vi "main.vi"(0 "Test Pins":T7, 1 "Caller Information":T11, 5 "Test Inputs":T8={"Load Current in A"=0.0, "Input Voltage in V"=[], "Nominal Output Voltage in V"=0.0, "Required Vout drop"=0.1, "Advance Setting"={"Prepare"={"Load SMU Output Function"=enum."VoltageSource"}, "Stimulus and Measure"={"Loop Delay in milliseconds"=1}}}, 11 "error in":errorcluster) -> (4 "Test Results":T14 {"Measured Input Voltage in V" format="%#.5g"; "Dropout Voltage in V" format="%#.5g"; "Measured Output Voltage in V" format="%#.5g"}, 15 "error out":errorcluster)   [LabVIEW 2020, in "LDO Dropout Voltage.lvlib"]
doc: "<b>Caller</b> Information is input for framework components. Mode should be set to <b>Automation</b> when running from TestStand. Sequence Context should be set to <b>ThisContext</b> when running from TestStand. The values will be updated everytime the setting is applied using \"Edit\" dialog.\n\n<b>Test Pins</b> is names of pins available in the pinmap file. Provide the right pins for the required functionality.\n\n<b>Test Inputs</b> is input required for the measurement to perform.\n\n<b>error in</b> is meant for the sequencing. <b>error in</b> should be <b>no error</b> always.\n\n<b>Test Results</b> contains all the measured data during the measurement and processed results.\n\n<b>error out</b> contains the error occured during measurement.\n\nCheck measurement documentation for more information (<Program Files>\\Soliton Technologies\\MeasurementSuite\\CodeModules\\LDO\\LDO Dropout Voltage.pdf)"
uses:
  LDO Dropout Voltage.lvlib
  Typedefs/Test Results.ctl
  Typedefs/Test Inputs.ctl
  Typedefs/Advance Settings.ctl
  Reusables/Instrument APIs/Load Output Function.ctl
  <userlib>/_Soliton/Measurement Suite/Reusables/Plugin Common/Typedefs/Caller Events.ctl
  <userlib>/_Soliton/Measurement Suite/Reusables/Plugin Common/Typedefs/Caller Information.ctl
  <userlib>/_Soliton/Measurement Suite/Reusables/Plugin Common/Typedefs/Caller Mode.ctl
  Typedefs/Test Pins.ctl
  Typedefs/Pin Dropdown.ctl
  <userlib>/_Soliton/Measurement Suite/Reusables/Plugin Common/Typedefs/Termination Monitor Info.ctl
  <vilib>/Utility/miscctls.llb/LVAnnotationListTypeDef.ctl
  <vilib>/Utility/error.llb/DialogType.ctl
  dc46d5cc-eb00-4f7e-b59b-e7fbb9f2ed4c.vi
  f0cc231b-6294-4813-9d5b-a7ddc5043ff2.vi
  f8cfc4b9-01f6-4b8f-8ca0-5ef2fe22dc8a.vi
  be024a05-4f6c-4aec-bf2b-5f4e194505bf.vi
  6ac4b11f-8d38-44bc-9b0c-66f4c353a8b6.vi
  bb3e62c4-a2c2-4505-9438-f842dd651d6c.vi
  ce2ee1e5-697c-4608-b941-8c9b0f21ffd9.vi
  0b250ff7-52ee-4af6-80b1-a8d503da2759.vi
  6a7d4b92-ccd7-4b01-a579-e3d7f201896e.vi
  <userlib>/_Soliton/Measurement Suite/Reusables/InstrumentSessionAPIs/SessionManagerApiPath.vi
  <vilib>/Utility/sysdir.llb/Get System Directory.vi
  <vilib>/Utility/LVLibp/Get Exported File Path.vi
  <userlib>/_Soliton/Measurement Suite/Reusables/Errors/Error 6001.vi
  <userlib>/_Soliton/Measurement Suite/Reusables/Plugin Common/Plugin Common.lvlib
  <userlib>/_Soliton/Measurement Suite/Reusables/Queue Driver/Plugin Queue Driver.lvlib
panel:
  out "Progress":i32(slide) scale=-1.0..5.0
  in  "Terminate":bool
  in  "Run":bool caption="Measure"
  in  "Exit":bool
  out "Header":string
  in  "Tab Enum":T1(radio)
  out "Tab Control":T2(tab)
  in  "SystemSetup":T4={"Set Input Voltage"={"PinStatus"=0, "PinName"="", "Info"=TRUE}, "Measure Input Voltage"={"PinStatus"=0, "PinName"="", "Info"=TRUE}, "Set Load Current"={"PinStatus"=0, "PinName"="", "Info"=TRUE}, "Measure Output Voltage"={"PinStatus"=0, "PinName"="", "Info"=TRUE}}
  in  "Req. Voltage Drop":dbl=0.1 caption="Required drop in Output Voltage (V)" format="%#_6p"
  in  "Step Input":T5 {"Step Size (V)" min=0.0 format="%#_6p"; "Stop Value (V)" format="%#_6p"; "Start Value (V)" format="%#_6p"}
  in  "Customize Sweep Value":bool
  in  "Input Voltage (V)":dbl[](array[numeric]) format="%#_6p"
  in  "Nominal Output Voltage (V)":dbl format="%#_6p"
  in  "Customize Sweep Value":enum32{"Item 0", "Item 1"}(radio)
  in  "Load Current (A)":dbl format="%#_6p"
  in  "Advanced Settings":bool
  out "Result Tab":T6(tab)
  out "Dropout Voltage":cluster{"Iload (mA)":dbl[], "Vout (V)":dbl[]}(graph)
  out "Measured Values":string[][](table)
  out "Dropout Voltage (V)":dbl format="%#.5p"
  in  "Result Enum":T6(radio)
  in  "ErrorOccured":errorcluster
  in  "DataLogPath":path
  in  "Caller Events":T13
  # "Supports NIDmmInstrument"
  # "Supports NIDmmInstrument"
  # "Supports NIDCPowerInstrument"
  # "Supports NIDCPowerInstrument"
  # "Fill Input Voltage list using the following"
  # "Dropout Voltage Calculation"
  # "Vdropout = Input Voltage_x - Output Voltage_x\n\nIn the other words, Vdropout = Input Voltage - Output Voltage,\nwhen the Output Voltage has decreased from Output Voltage_Nominal by Required drop in Output Voltage"
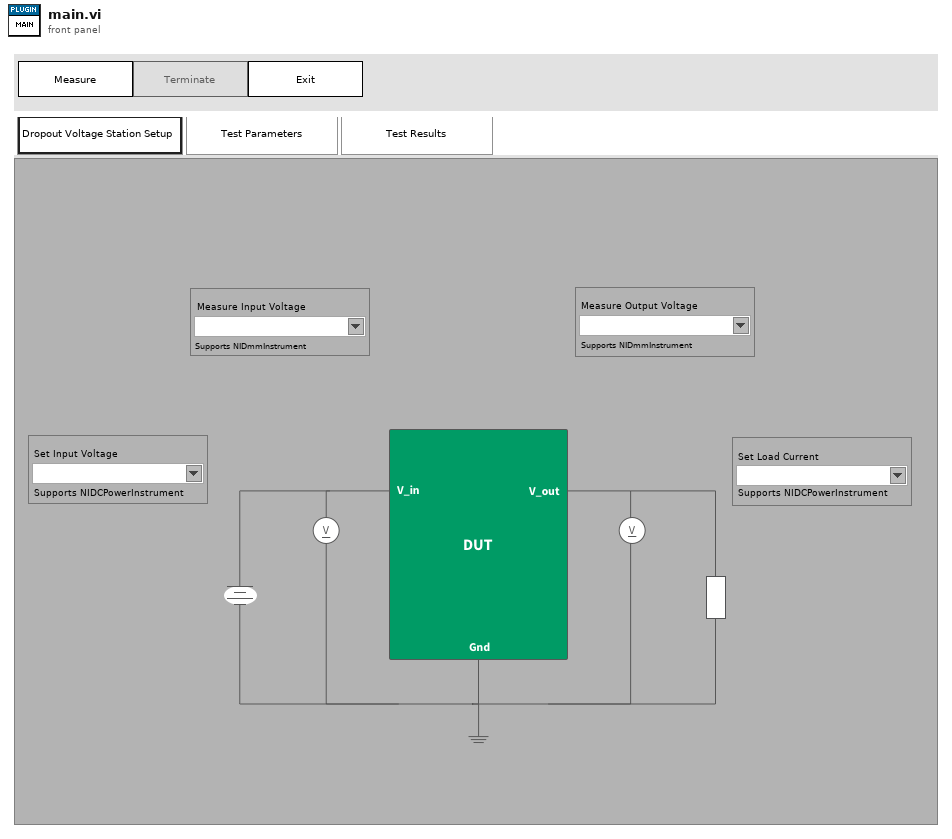
[diagram p1: front panel]
types:
  T1 = enum32{"Station Setup", "Test Parameters", "Test Results"}
  T2 = enum32{"Station Setup", "Test Parameters", "Test Results", "Debug"}
  T3 = typedef "LDO Dropout Voltage.lvlib/Pin Dropdown.ctl" = cluster{"PinStatus":u16, "PinName":string, "Info":bool}
  T4 = cluster{"Set Input Voltage":T3, "Measure Input Voltage":T3, "Set Load Current":T3, "Measure Output Voltage":T3}
  T5 = cluster{"Start Value (V)":dbl, "Stop Value (V)":dbl, "Step Size (V)":dbl}
  T6 = enum32{"Output Voltage Vs Input Voltage Curve", "Measured Value Table View"}
  T7 = typedef "LDO Dropout Voltage.lvlib/Test Pins.ctl" = cluster{"Set Input Voltage":string, "Measure Input Voltage":string, "Set Load Current":string, "Measure Output Voltage":string}
  T8 = typedef "LDO Dropout Voltage.lvlib/Test Inputs.ctl" = cluster{"Load Current in A":dbl, "Input Voltage in V":dbl[], "Nominal Output Voltage in V":dbl, "Required Vout drop":dbl, "Advance Setting":T9}
  T9 = typedef "LDO Dropout Voltage.lvlib/Advance Settings.ctl" = cluster{"Prepare":cluster{"Load SMU Output Function":T10}, "Stimulus and Measure":cluster{"Loop Delay in milliseconds":u32}}
  T10 = typedef "Load Output Function.ctl" = enum16{"VoltageSource", "CurrentSource"}
  T11 = typedef "Plugin Common.lvlib/Caller Information.ctl" = cluster{"Mode":T12, "Sequence Context":refnum<k7>}
  T12 = typedef "Caller Mode.ctl" = enum16{"Standalone", "Automation", "MeasurementSuite"}
  T13 = typedef "Plugin Common.lvlib/Caller Events.ctl" = cluster{"Caller Event":refnum<user-event>}
  T14 = typedef "LDO Dropout Voltage.lvlib/Test Results.ctl" = cluster{"Measured Input Voltage in V":dbl[], "Measured Output Voltage in V":dbl[], "Dropout Voltage in V":dbl}
  T15 = typedef "Plugin Common.lvlib/Termination Monitor Info.ctl" = cluster{"Caller Information":T11, "Execution":refnum<k7>, "Termination Monitor":refnum<k7>, "Type":string, "Plugin Name":string}
  T16 = cluster{"Termination Monitor Info":T15, "Test Inputs":T8, "Test Results":T14, "Test Results[][]":string[][], "Test Pins":T7, "Logger Folder Path":path, "Valid Logger Path?":bool, "Logger File Path":path, "UI Ctls":refnum<vi>[], "Input Voltage_x":dbl, "Output Voltage_x":dbl}
  T17 = enum8{"Enabled", "Disabled", "Disabled and Grayed Out"}
  T18 = cluster{"Name":string, "Color":u32, "Style":u8, "Point Style":u8, "Name Visible":bool, "Allow Drag":bool, "Cursor Mode":u32, "Plot":i32, "Index":i32, "Position":cluster{"X":dbl, "Y":dbl}, "X Scale":u32, "Y Scale":u32, "Watch Plots":i32[], "Watch All Plots":bool, "Plot Area":i32, "Label Offset":cluster{"X":dbl, "Y":dbl}}
  T19 = typedef "LVAnnotationListTypeDef.ctl" = cluster{"Name":string, "Color":u32, "Style":u8, "Point Style":u8, "Name Visible":bool, "Allow Drag":bool, "Annotation Mode":u32, "Plot":i32, "Index":i32, "Position":cluster{"X":dbl, "Y":dbl}, "X Scale":u32, "Y Scale":u32, "Show Arrow":bool, "Lock Name":bool, "Plot Area":i32, "Label Offset":cluster{"X":dbl, "Y":dbl}}[]
  T20 = cluster{"Start Value":dbl, "Stop Value":dbl, "Step Size":dbl}
  T21 = typedef "LVCursorListTypeDef.ctl" = cluster{"Name":string, "Color":u32, "Style":u8, "Point Style":u8, "Name Visible":bool, "Allow Drag":bool, "Cursor Mode":u32, "Plot":i32, "Index":i32, "Position":cluster{"X":dbl, "Y":dbl}, "X Scale":u32, "Y Scale":u32, "Watch Plots":i32[], "Watch All Plots":bool, "Plot Area":i32, "Label Offset":cluster{"X":dbl, "Y":dbl}}[]
  T22 = cluster{"Name":string, "Color":u32, "Style":u8, "Point Style":u8, "Name Visible":bool, "Allow Drag":bool, "Annotation Mode":u32, "Plot":i32, "Index":i32, "Position":cluster{"X":dbl, "Y":dbl}, "X Scale":u32, "Y Scale":u32, "Show Arrow":bool, "Lock Name":bool, "Plot Area":i32, "Label Offset":cluster{"X":dbl, "Y":dbl}}
  T23 = cluster{"Measured Input Voltage in V":dbl[], "Measured Output Voltage in V":dbl[]}
  T24 = typedef "DialogType.ctl" = u16
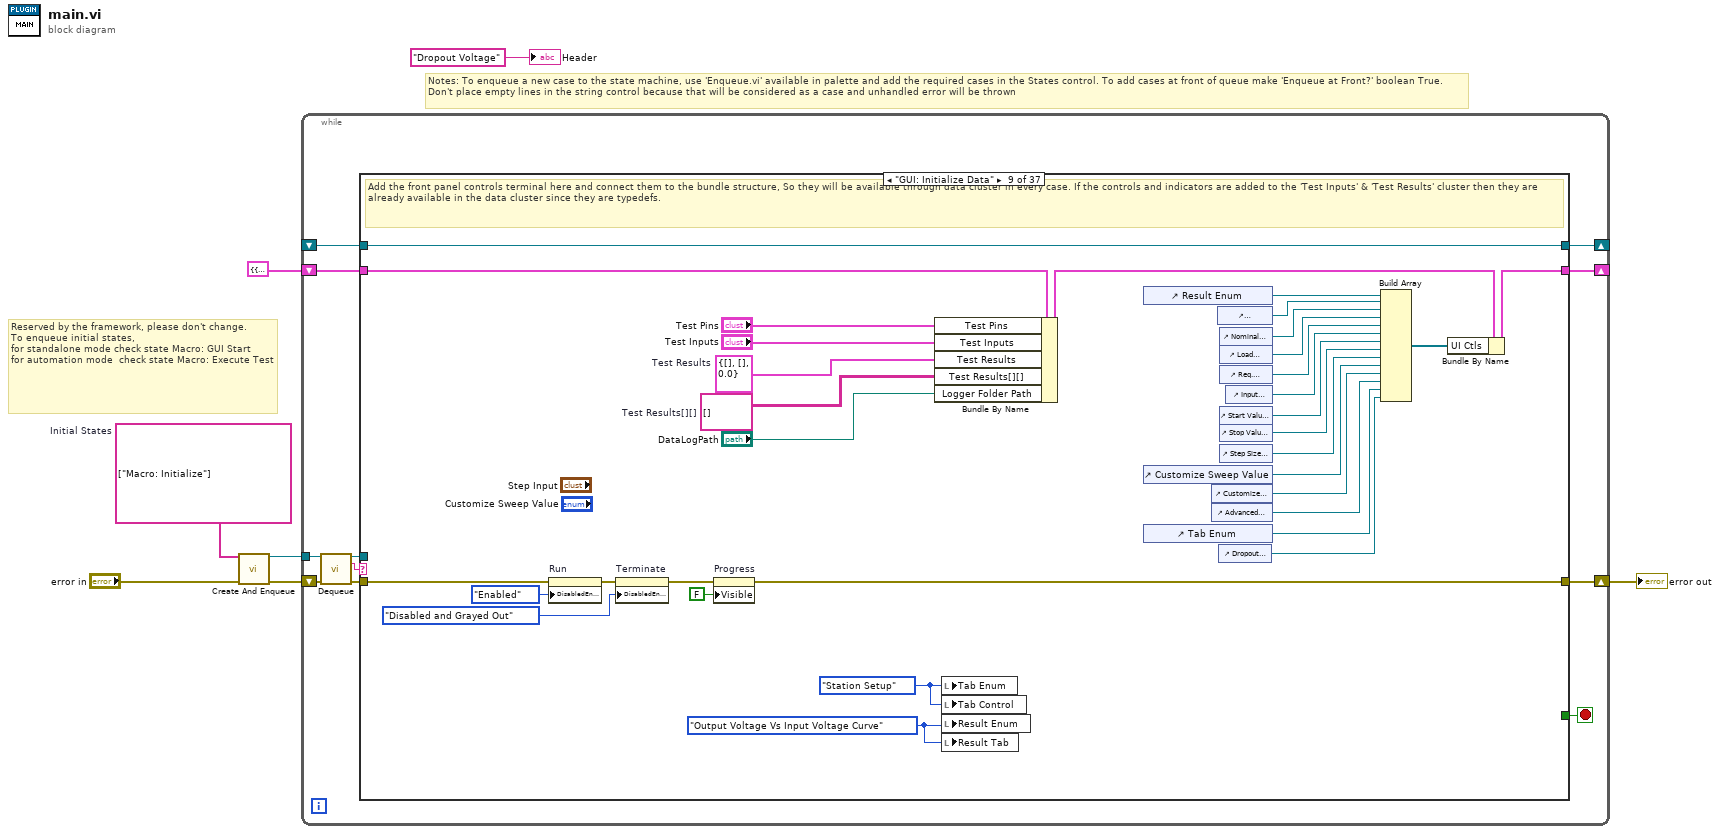
[diagram p0: block diagram]
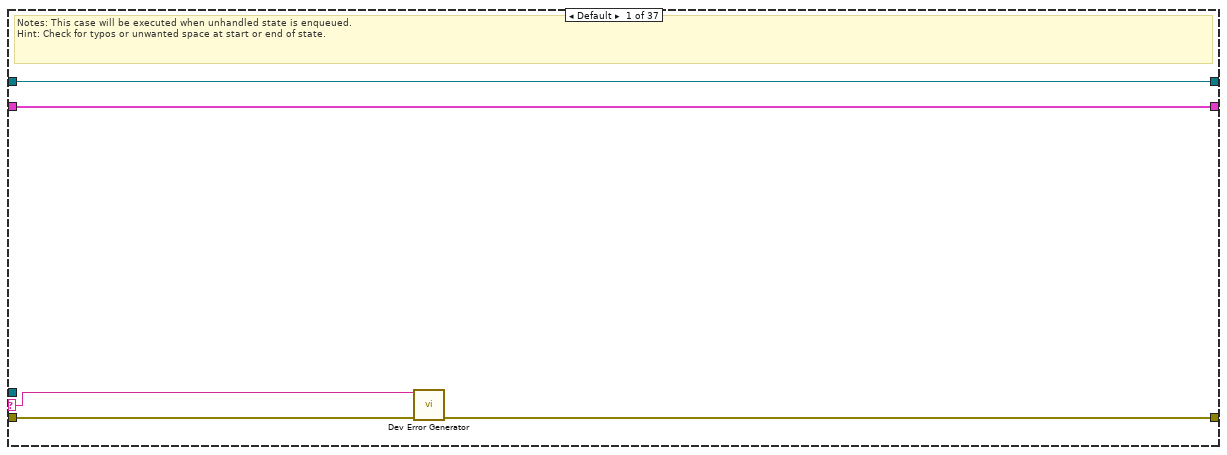
[diagram p2: hidden frame]
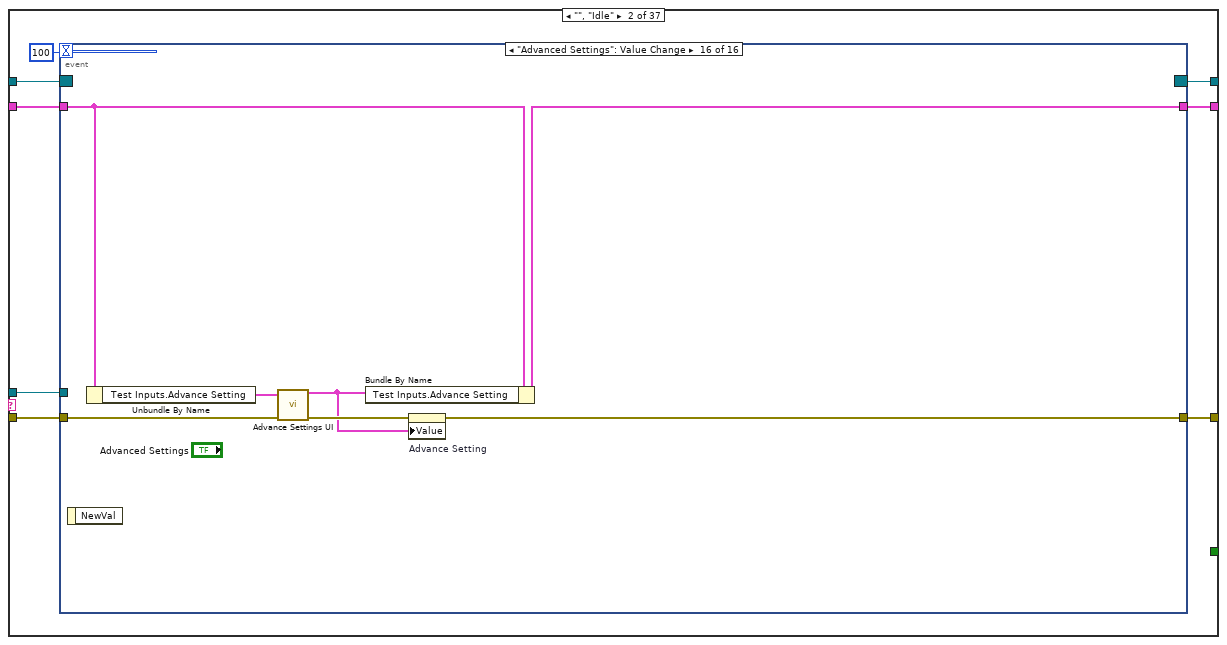
[diagram p3: hidden frame]
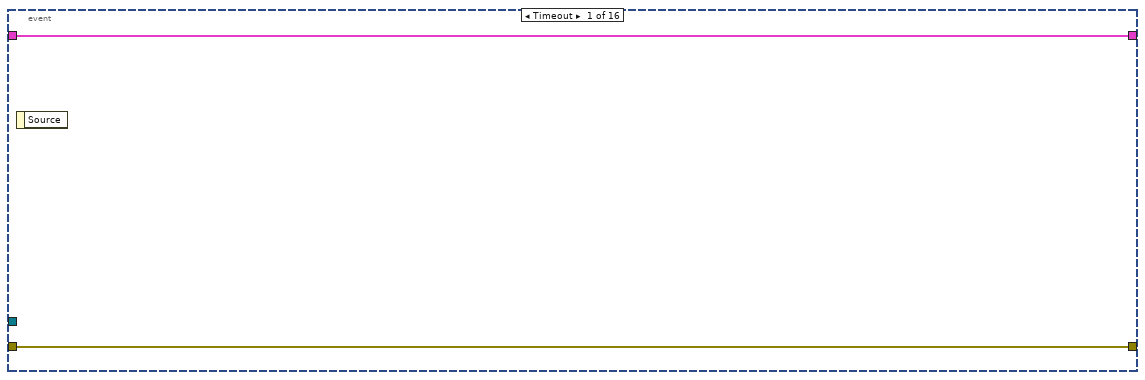
[diagram p4: hidden frame]
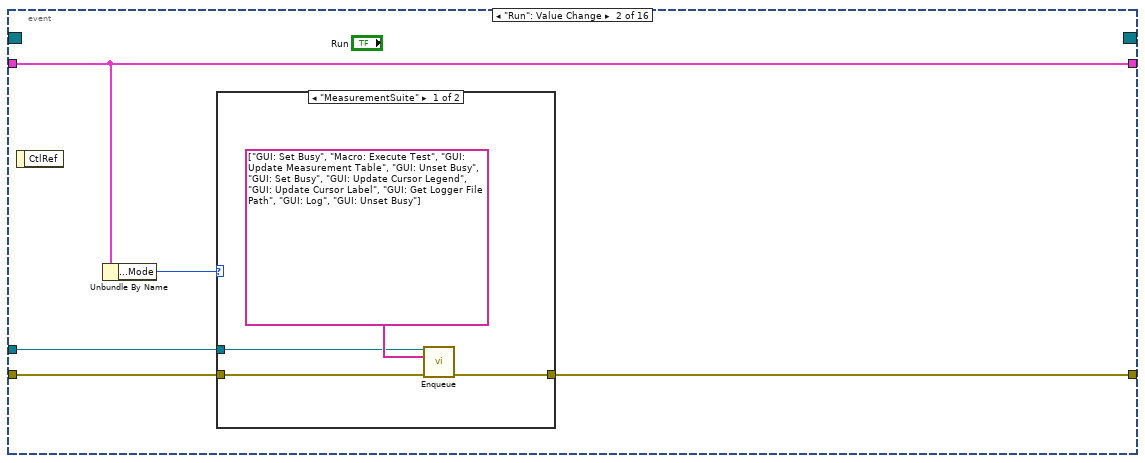
[diagram p5: hidden frame]
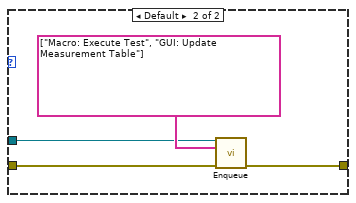
[diagram p6: hidden frame]
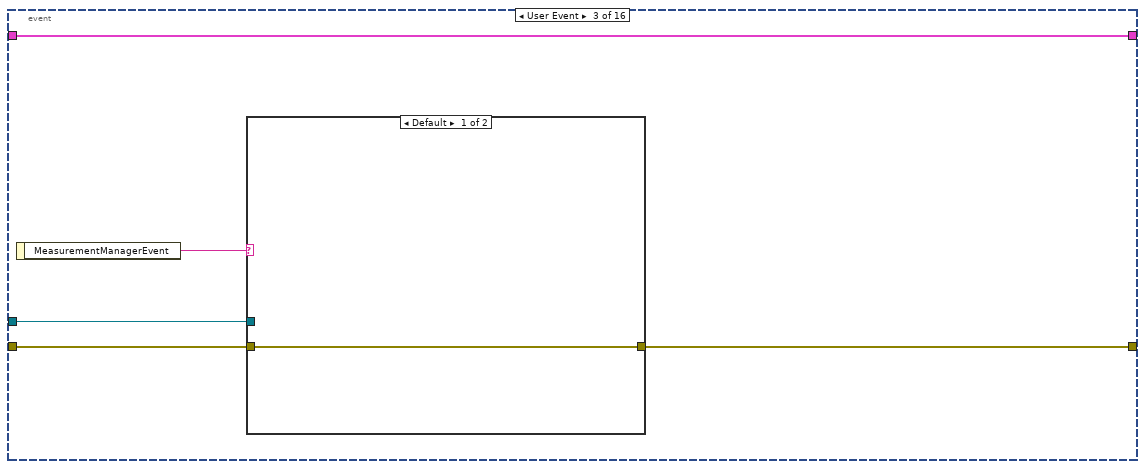
[diagram p7: hidden frame]
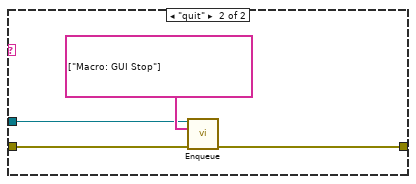
[diagram p8: hidden frame]
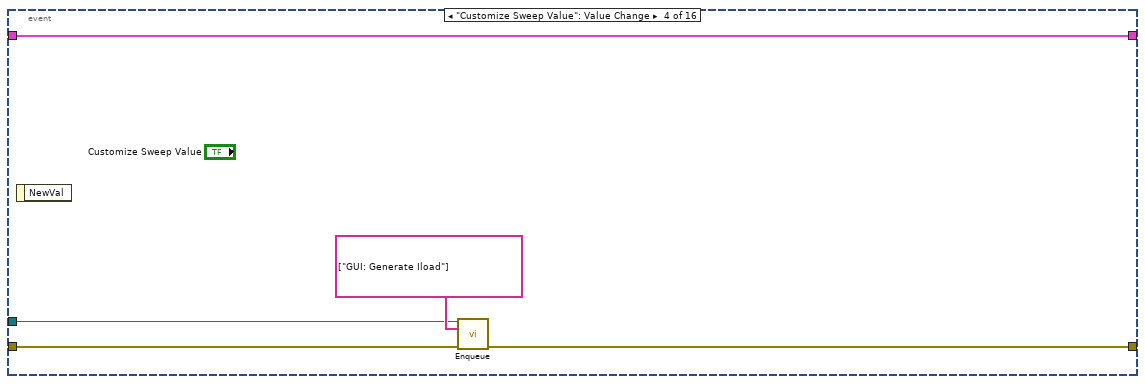
[diagram p9: hidden frame]
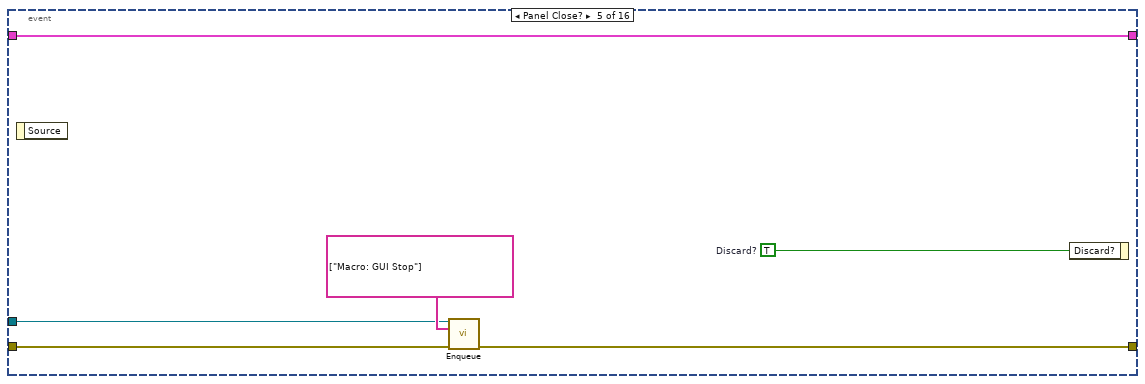
[diagram p10: hidden frame]
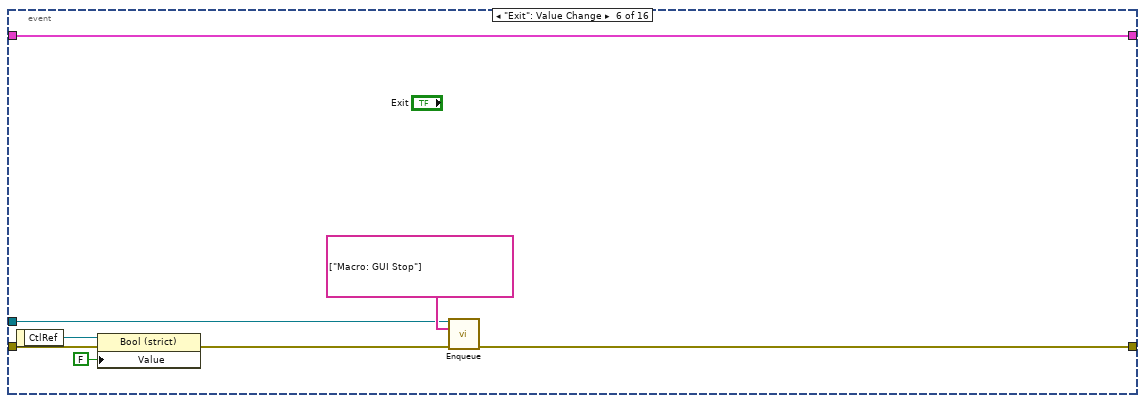
[diagram p11: hidden frame]
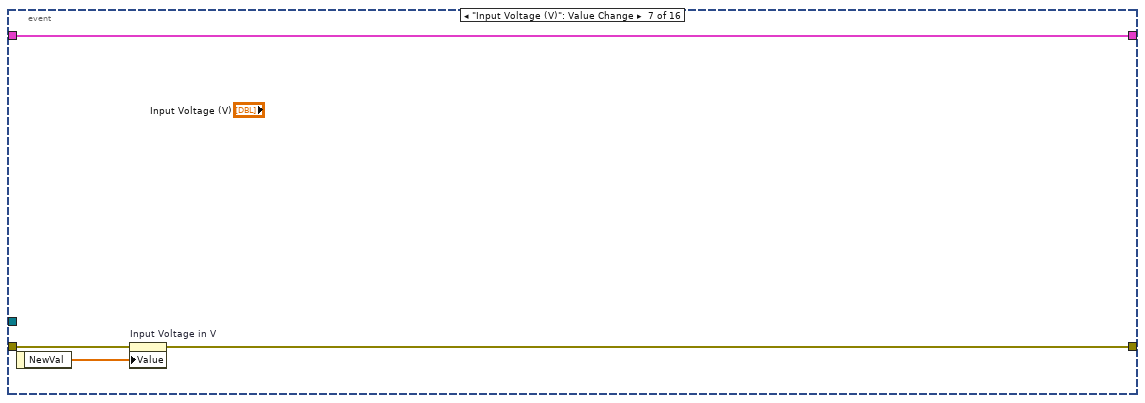
[diagram p12: hidden frame]
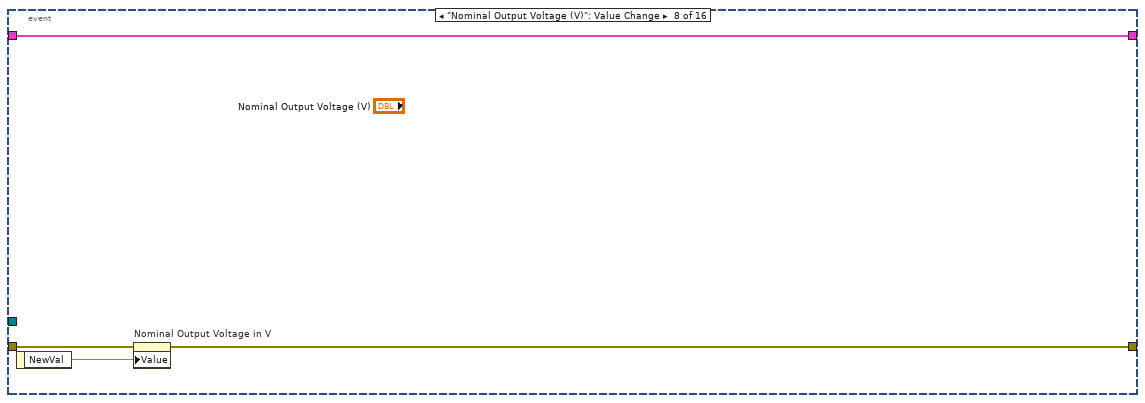
[diagram p13: hidden frame]
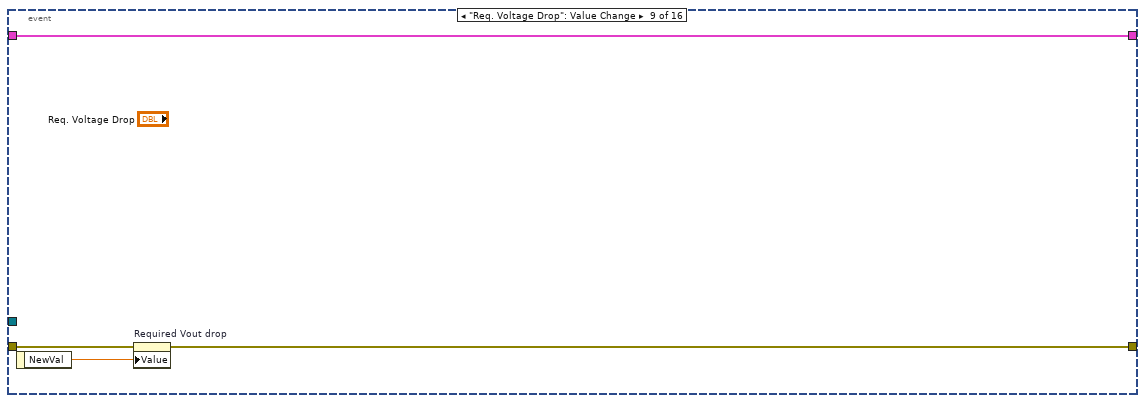
[diagram p14: hidden frame]
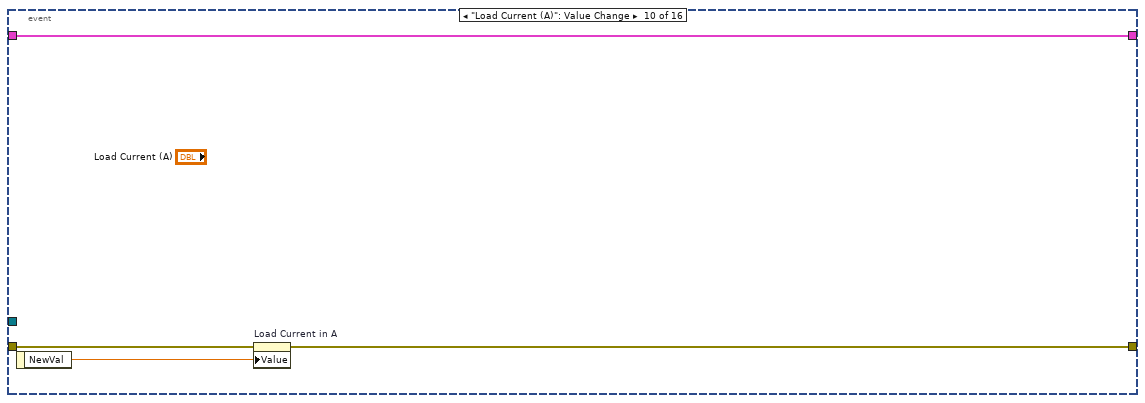
[diagram p15: hidden frame]
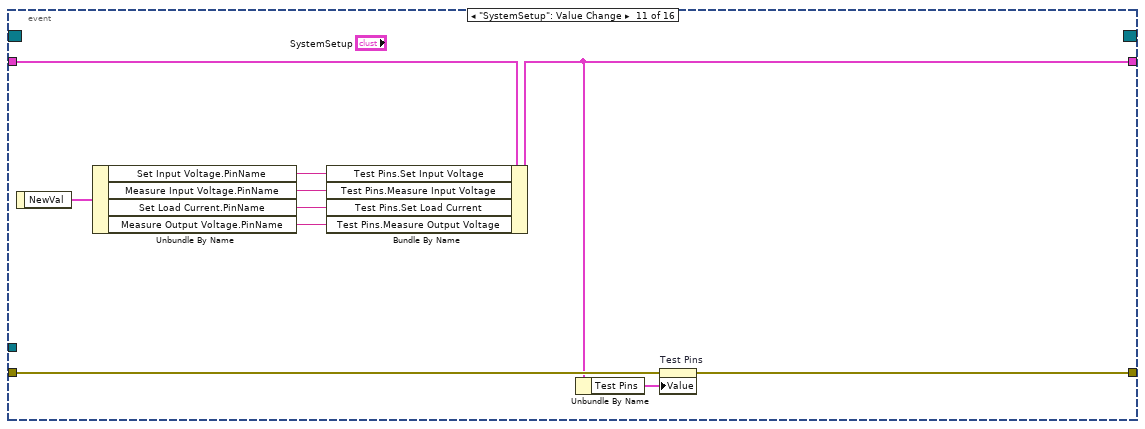
[diagram p16: hidden frame]
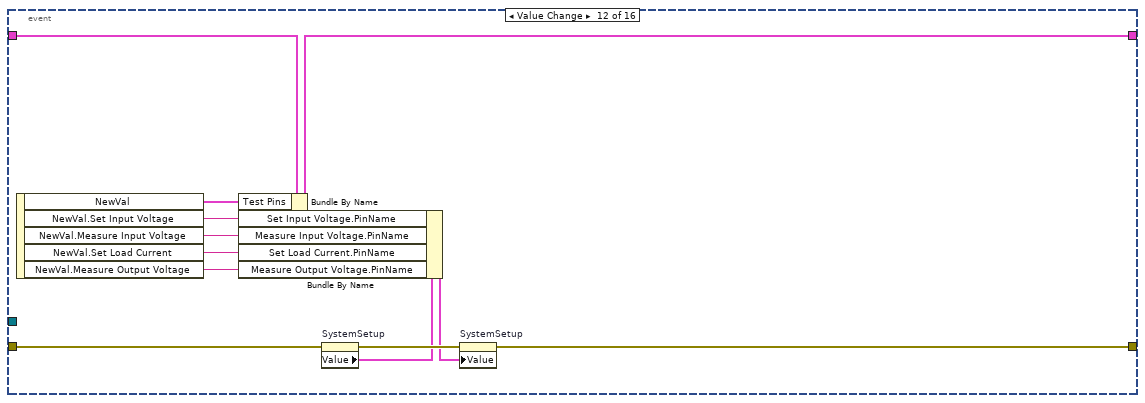
[diagram p17: hidden frame]
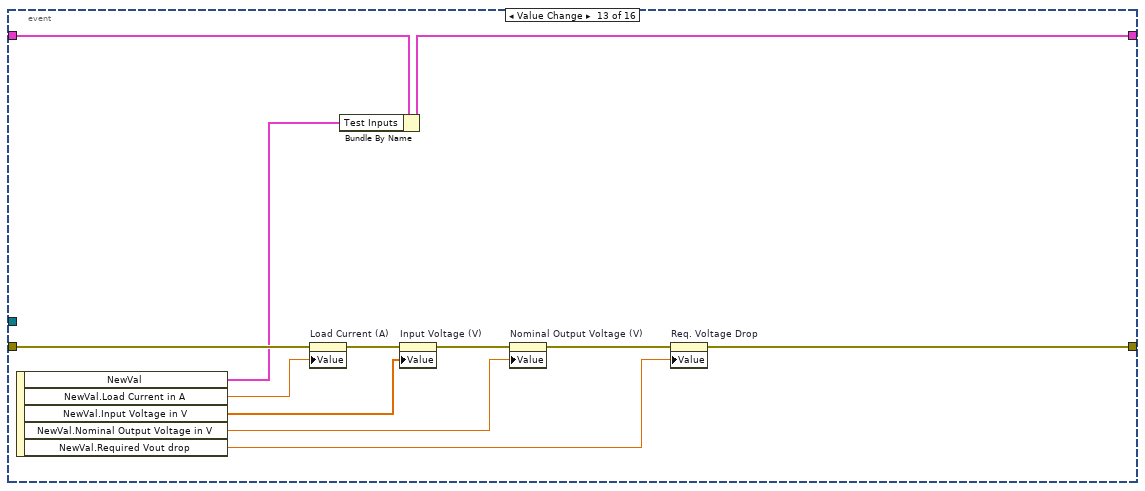
[diagram p18: hidden frame]
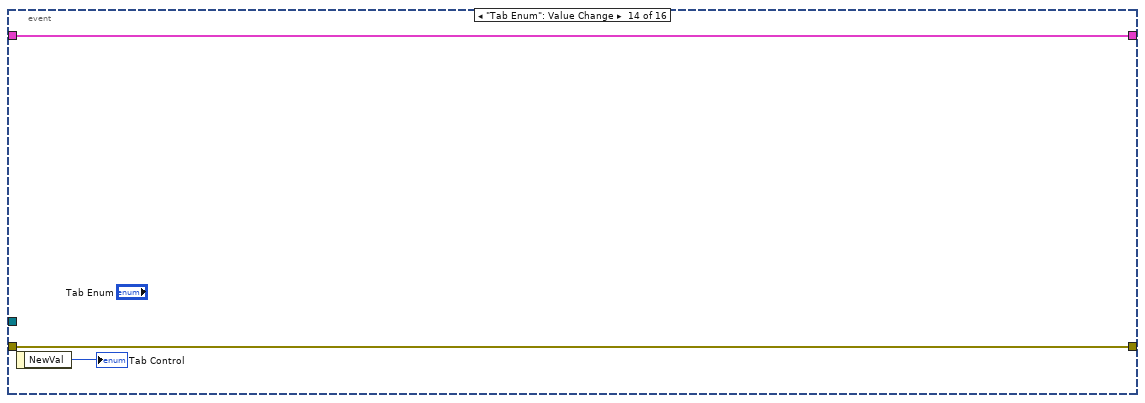
[diagram p19: hidden frame]
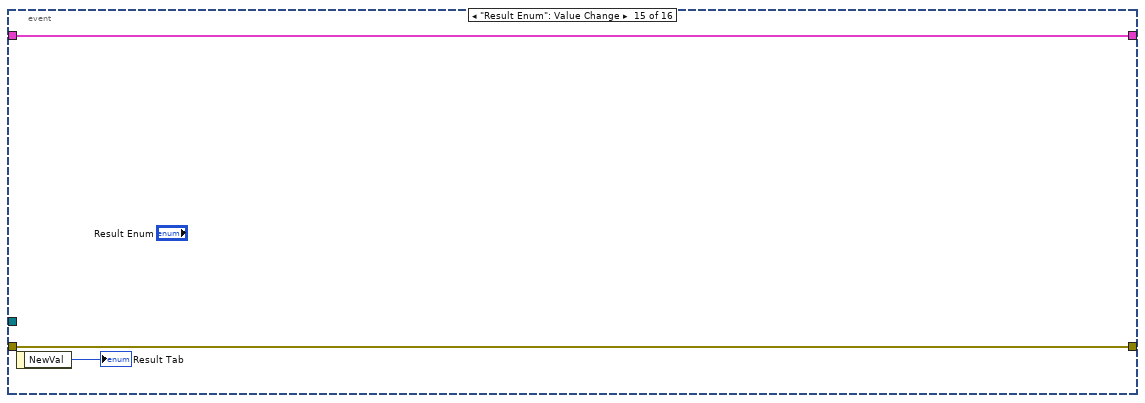
[diagram p20: hidden frame]
diagram:
  w7 = string[] ["Macro: Initialize"]  # Initial States
  # "Notes: To enqueue a new case to the state machine, use 'Enqueue.vi' available in palette and add the required cases in the States control. To add cases at front of queue make 'Enqueue at Front?' boolean True. Don't place empty lines in the string control because that will be considered as a case and unhandled error will be thrown"
  # "Reserved by the framework, please don't change. \nTo enqueue initial states,\nfor standalone mode check state Macro: GUI Start\nfor automation mode  check state Macro: Execute Test"
  n1 = call <userlib>:"Create And Enqueue.vi"("Initial States"=w7, "error in (no error)"="error in") -> ("Queue out"=w5:refnum<queue>, "error out"=w3:errorcluster)  [unwired: 12 in]
  n2 = while {
    shift-right: [w18] -> w4
    shift-left: w3 -> [w16]
    shift-right: [w14] -> _
    shift-left: T16 {"Termination Monitor Info"={"Caller Information"={"Mode"=enum."Standalone", "Sequence Context"=refnum}, "Execution"=refnum, "Termination Monitor"=refnum, "Type"="", "Plugin Name"=""}, "Test Inputs"={"Load Current in A"=0.0, "Input Voltage in V"=[], "Nominal Output Voltage in V"=0.0, "Required Vout drop"=0.0, "Advance Setting"={"Prepare"={"Load SMU Output Function"=enum."VoltageSource"}, "Stimulus and Measure"={"Loop Delay in milliseconds"=0}}}, "Test Results"={"Measured Input Voltage in V"=[], "Measured Output Voltage in V"=[], "Dropout Voltage in V"=0.0}, "Test Results[][]"=[], "Test Pins"={"Set Input Voltage"="", "Measure Input Voltage"="", "Set Load Current"="", "Measure Output Voltage"=""}, "Logger Folder Path"=path "", "Valid Logger Path?"=FALSE, "Logger File Path"=path "", "UI Ctls"=[], "Input Voltage_x"=0.0, "Output Voltage_x"=0.0} -> [w13]
    tunnel: w5 -> [w12]
    shift-right: [w9] -> _
    shift-left: _ -> [w10]
    stop <- w17 stop-if-true
    n3 = call <userlib>:"Dequeue.vi"("Queue in"=w12, "error in (no error)"=w16) -> ("Queue out"=w11:refnum<queue>, "Dequeued State"=w8:string, "error out"=w15:errorcluster)  [unwired: 11 in]
    n4 = case shown="\"GUI: Initialize Data\"" w8 {
      selector: w8 -> [w21 _ _ _ _ _ _ _ _ _ _ _ _ _ _ _ _ _ _ _ _ _ _ _ _ _ _ _ _ _ _ _ _ _ _ _ _]
      tunnel: w15 -> [w20 w28 w141 w150 w159 w166 w173 w178 w204 w216 w220 w223 w238 w256 w268 w337 w341 w358 w369 w381 w396 w401 w408 w413 w426 w439 w457 w466 w479 w520 w533 w547 w558 w564 w572 w579 w597]
      tunnel: [w22 w29 w141 w153 w160 w167 w174 w178 w202 w214 w218 w223 w232 w256 w265 w335 w340 w359 w370 w383 w396 w402 w409 w413 w420 w435 w450 w464 w484 w506 w525 w547 w558 w561 w572 w577 w591] -> w18
      tunnel: [_ _ _ _ _ _ _ _ _ _ _ _ _ _ _ _ _ _ _ _ _ _ _ _ _ _ _ _ _ _ _ _ _ _ _ w574 TRUE] -> w17
      tunnel: [w23 w31 w140 w143 w161 w168 w175 w177 w194 w215 w219 w222 w226 w250 w261 w329 w339 w360 w368 w382 w395 w400 w407 w412 w419 w440 w458 w465 w486 w522 w535 w548 w557 w569 w571 w576 w598] -> w14
      tunnel: w13 -> [w23 w30 w140 w154 w161 w168 w175 w177 w209 w215 w219 w222 w225 w249 w261 w329 w338 w360 w368 w382 w395 w399 w406 w412 w430 w440 w458 w465 w487 w522 w535 w549 w557 w569 w571 w576 w598]
      tunnel: w11 -> [_ w24 _ w152 w157 w164 w171 _ _ _ _ _ _ _ _ _ _ _ _ _ _ _ _ _ _ _ _ _ _ _ _ _ _ _ _ w573 w596]
      tunnel: w10 -> [w19 w26 w139 w151 w156 w163 w170 w176 w208 _ w217 w221 w239 w255 w267 w336 w346 w361 w376 w389 w394 w403 w410 w411 w428 w441 w460 w467 w485 w523 w536 w550 w556 w568 w570 w578 w595]
      tunnel: [w19 w25 w139 w151 w156 w163 w170 w176 w208 w213 w217 w221 w239 w255 w267 w336 w346 w361 w376 w389 w394 w403 w410 w411 w428 w441 w460 w467 w485 w523 w536 w550 w556 w568 w570 w578 w595] -> w9
      frame Default {
        # "Notes: This case will be executed when unhandled state is enqueued. \nHint: Check for typos or unwanted space at start or end of state."
        n5 = call <userlib>:"Dev Error Generator.vi"("State"=w21, "error in (no error)"=w20) -> ("error out"=w22:errorcluster)  [unwired: 13 in]
      }
      frame "", "Idle" {
        n6 = event shown="[15] \"Advanced Settings\": Value Change" {
          selector: w26 -> [_ _ _ _ _ _ _ _ _ _ _ _ _ _ _ _]
          dyn-events: [_ _ _ _ _ _ _ _ _ _ _ _ _ _ _ _] -> w25
          timeout: 100 -> [_ _ _ _ _ _ _ _ _ _ _ _ _ _ _ _]
          tunnel: [w33 w35 w51 w61 w67 w75 w76 w83 w87 w91 w93 w108 w117 w128 w131 w135] -> w31
          tunnel: w30 -> [w33 w35 w51 w61 w67 w75 w76 w83 w87 w91 w97 w107 w116 w128 w131 w134]
          tunnel: [w32 w38 w49 w59 w64 w73 w78 w82 w86 w90 w95 w111 w115 w127 w130 w133] -> w29
          tunnel: w28 -> [w32 w37 w50 w58 w63 w72 w79 w81 w85 w89 w94 w113 w121 w127 w130 w137]
          tunnel: w24 -> [_ w36 w47 w57 w62 w71 _ _ _ _ _ _ _ _ _ _]
          event Timeout {
            n7 = event-data() -> ()  [unwired: 1 in, 1 out]
          }
          event "Run": Value Change {
            n8 = event-data() -> ()  [unwired: 1 in, 1 out]
            n9 = Unbundle By Name(w35) -> ("Termination Monitor Info.Caller Information.Mode"=w34:T12)
            n10 = case shown="\"MeasurementSuite\"" w34 {
              tunnel: [w41 w45] -> w38
              tunnel: w37 -> [w40 w44]
              tunnel: w36 -> [w39 w43]
              frame "MeasurementSuite" {
                n11 = call <userlib>:"Enqueue.vi"("Queue in"=w39, "States"=string[] ["GUI: Set Busy", "Macro: Execute Test", "GUI: Update Measurement Table", "GUI: Unset Busy", "GUI: Set Busy", "GUI: Update Cursor Legend", "GUI: Update Cursor Label", "GUI: Get Logger File Path", "GUI: Log", "GUI: Unset Busy"], "error in (no error)"=w40) -> ("error out"=w41:errorcluster)  [unwired: 11 in, 1 out]
              }
              frame Default {
                n12 = call <userlib>:"Enqueue.vi"("Queue in"=w43, "States"=string[] ["Macro: Execute Test", "GUI: Update Measurement Table"], "error in (no error)"=w44) -> ("error out"=w45:errorcluster)  [unwired: 11 in, 1 out]
              }
            }
          }
          event User Event {
            n13 = event-data() -> ("MeasurementManagerEvent"=w48:string)  [unwired: 1 in]
            n14 = case shown="Default" w48 {
              tunnel: [w52 w53] -> w49
              tunnel: w50 -> [w52 w55]
              tunnel: w47 -> [_ w54]
              frame Default {
              }
              frame "quit" {
                n15 = call <userlib>:"Enqueue.vi"("Queue in"=w54, "States"=string[] ["Macro: GUI Stop"], "error in (no error)"=w55) -> ("error out"=w53:errorcluster)  [unwired: 11 in, 1 out]
              }
            }
          }
          event "Customize Sweep Value": Value Change {
            n16 = event-data() -> ()  [unwired: 1 in, 1 out]
            n17 = call <userlib>:"Enqueue.vi"("Queue in"=w57, "States"=string[] ["GUI: Generate Iload"], "error in (no error)"=w58) -> ("error out"=w59:errorcluster)  [unwired: 11 in, 1 out]
          }
          event Panel Close? {
            w66 = TRUE  # Discard?
            n18 = event-data() -> ()  [unwired: 1 in, 1 out]
            n19 = call <userlib>:"Enqueue.vi"("Queue in"=w62, "States"=string[] ["Macro: GUI Stop"], "error in (no error)"=w63) -> ("error out"=w64:errorcluster)  [unwired: 11 in, 1 out]
            n20 = event-data("Discard?"=w66) -> ()  [unwired: 1 in, 1 out]
          }
          event "Exit": Value Change {
            n21 = event-data() -> ("CtlRef"=w69:refnum<vi>)  [unwired: 1 in]
            n22 = property class="Bool (strict)"(reference=w69, error in=w72, "Value"=FALSE) -> (error out=w70:errorcluster)  [unwired: 1 out]
            n23 = call <userlib>:"Enqueue.vi"("Queue in"=w71, "States"=string[] ["Macro: GUI Stop"], "error in (no error)"=w70) -> ("error out"=w73:errorcluster)  [unwired: 11 in, 1 out]
          }
          event "Input Voltage (V)": Value Change {
            n24 = event-data() -> ("NewVal"=w77:dbl[])  [unwired: 1 in]
            n25 = property on="Input Voltage in V" class="Arr (strict)"(error in=w79, "Value"=w77) -> (error out=w78:errorcluster)  [unwired: 1 in, 1 out]
          }
          event "Nominal Output Voltage (V)": Value Change {
            n26 = event-data() -> ("NewVal"=w80:dbl)  [unwired: 1 in]
            n27 = property on="Nominal Output Voltage in V" class="DigNum (strict)"(error in=w81, "Value"=w80) -> (error out=w82:errorcluster)  [unwired: 1 in, 1 out]
          }
          event "Req. Voltage Drop": Value Change {
            n28 = event-data() -> ("NewVal"=w84:dbl)  [unwired: 1 in]
            n29 = property on="Required Vout drop" class="DigNum (strict)"(error in=w85, "Value"=w84) -> (error out=w86:errorcluster)  [unwired: 1 in, 1 out]
          }
          event "Load Current (A)": Value Change {
            n30 = event-data() -> ("NewVal"=w88:dbl)  [unwired: 1 in]
            n31 = property on="Load Current in A" class="DigNum (strict)"(error in=w89, "Value"=w88) -> (error out=w90:errorcluster)  [unwired: 1 in, 1 out]
          }
          event "SystemSetup": Value Change {
            n32 = event-data() -> ("NewVal"=w96:T4)  [unwired: 1 in]
            n33 = Unbundle By Name(w96) -> ("Set Input Voltage.PinName"=w101:string, "Measure Input Voltage.PinName"=w100:string, "Set Load Current.PinName"=w99:string, "Measure Output Voltage.PinName"=w98:string)
            n34 = Bundle By Name(cluster=w97, "Test Pins.Set Input Voltage"=w101, "Test Pins.Measure Input Voltage"=w100, "Test Pins.Set Load Current"=w99, "Test Pins.Measure Output Voltage"=w98) -> (w93:T16)
            n35 = Unbundle By Name(w93) -> ("Test Pins"=w92:T7)
            n36 = property on="Test Pins" class="Clust (strict)"(error in=w94, "Value"=w92) -> (error out=w95:errorcluster)  [unwired: 1 in, 1 out]
          }
          event Value Change {
            n37 = event-data() -> ("NewVal"=w102:T7, "NewVal.Set Input Voltage"=w106:string, "NewVal.Measure Input Voltage"=w105:string, "NewVal.Set Load Current"=w103:string, "NewVal.Measure Output Voltage"=w104:string)  [unwired: 1 in]
            n38 = Bundle By Name(cluster=w107, "Test Pins"=w102) -> (w108:T16)
            n39 = property on="SystemSetup" class="Clust (strict)"(error in=w113) -> (error out=w112:errorcluster, "Value"=w110:T4)  [unwired: 1 in, 1 out]
            n40 = Bundle By Name(cluster=w110, "Set Input Voltage.PinName"=w106, "Measure Input Voltage.PinName"=w105, "Set Load Current.PinName"=w103, "Measure Output Voltage.PinName"=w104) -> (w109:T4)
            n41 = property on="SystemSetup" class="Clust (strict)"(error in=w112, "Value"=w109) -> (error out=w111:errorcluster)  [unwired: 1 in, 1 out]
          }
          event Value Change {
            n42 = event-data() -> ("NewVal"=w118:T8, "NewVal.Load Current in A"=w119:dbl, "NewVal.Input Voltage in V"=w124:dbl[], "NewVal.Nominal Output Voltage in V"=w122:dbl, "NewVal.Required Vout drop"=w114:dbl)  [unwired: 1 in]
            n43 = property on="Load Current (A)" class="DigNum (strict)"(error in=w121, "Value"=w119) -> (error out=w120:errorcluster)  [unwired: 1 in, 1 out]
            n44 = Bundle By Name(cluster=w116, "Test Inputs"=w118) -> (w117:T16)
            n45 = property on="Input Voltage (V)" class="Arr (strict)"(error in=w120, "Value"=w124) -> (error out=w125:errorcluster)  [unwired: 1 in, 1 out]
            n46 = property on="Nominal Output Voltage (V)" class="DigNum (strict)"(error in=w125, "Value"=w122) -> (error out=w123:errorcluster)  [unwired: 1 in, 1 out]
            n47 = property on="Req. Voltage Drop" class="DigNum (strict)"(error in=w123, "Value"=w114) -> (error out=w115:errorcluster)  [unwired: 1 in, 1 out]
          }
          event "Tab Enum": Value Change {
            n48 = event-data() -> ("NewVal"=→"Tab Control":T1)  [unwired: 1 in]
          }
          event "Result Enum": Value Change {
            n49 = event-data() -> ("NewVal"=→"Result Tab":T6)  [unwired: 1 in]
          }
          event "Advanced Settings": Value Change {
            n50 = event-data() -> ()  [unwired: 1 in, 1 out]
            n51 = Unbundle By Name(w134) -> ("Test Inputs.Advance Setting"=w136:T9)
            n52 = call "Advance Settings UI.vi"("Advance Setting"=w136, "error in (no error)"=w137) -> ("Advance Setting Out"=w132:T9, "error out"=w138:errorcluster)  [unwired: 12 in]
            n53 = Bundle By Name(cluster=w134, "Test Inputs.Advance Setting"=w132) -> (w135:T16)
            n54 = property on="Advance Setting" class="Clust (strict)"(error in=w138, "Value"=w132) -> (error out=w133:errorcluster)  [unwired: 1 in, 1 out]
          }
        }
      }
      frame "----------------- Macro ---------------" {
        # "Not used. category splitter"
      }
      frame "Macro: Initialize" {
        w147 = string[] ["Macro: GUI Start"]  # Standalone: Start the debug
        w148 = string[] ["Macro: Execute Test", "Exit"]  # Automation: Execute and stop
        # "Hidden in UI"
        # "This case decides the mode of the execution. Debug Mode: The plugin will act as a standalone GUI where user can change inputs, run test and debug the system. automation mode: The plugin will act as a flat code and go through all the test procedures and stops."
        n55 = call <userlib>:"Get Mode.vi"("Caller Information"="Caller Information", "error in (no error)"=w150) -> ("Automation(F) \\ Standalone (T)"=w146:bool, "error out"=w149:errorcluster)  [unwired: 12 in]
        n56 = Bundle By Name(cluster=w154, "Termination Monitor Info.Caller Information"="Caller Information") -> (w143:T16)
        n57 = Select(t=w147, s=w146, f=w148) -> (s? t:f=w145:string[])
        n58 = call <userlib>:"Enqueue.vi"("Queue in"=w152, "States"=w145, "Enqueue at Front?(F)"=TRUE, "error in (no error)"=w149) -> ("error out"=w153:errorcluster)  [unwired: 10 in, 1 out]
      }
      frame "Macro: Execute Test" {
        w158 = string[] ["TerminationMonitor: Start", "Test: Start", "Test: Prepare DCPower", "Test: Prepare DMM", "Test: Set Load Current", "Test: Sweep Over Voltage", "Test: Cleanup DCPower", "Test: Cleanup DMM", "Test: Calculate Dropout Voltage", "Test: Update UI", "Test: End", "TerminationMonitor: Stop"]  # Test Procedure
        # "List the states required for the test procedure. This state will be called in both automation mode and standalone mode when requested to run the test.\nDont remove 'Test: Start' and 'Test: End'."
        n59 = call <userlib>:"Enqueue.vi"("Queue in"=w157, "States"=w158, "Enqueue at Front?(F)"=TRUE, "error in (no error)"=w159) -> ("error out"=w160:errorcluster)  [unwired: 10 in, 1 out]
      }
      frame "Macro: GUI Start" {
        # "Initialize the data cluster for the standalone mode and register for the event from caller.\nDon't remove 'GUI: Initialize Data' and 'GUI: Register Event'."
        n60 = call <userlib>:"Enqueue.vi"("Queue in"=w164, "States"=string[] ["GUI: Initialize Data", "GUI: Register Event"], "Enqueue at Front?(F)"=TRUE, "error in (no error)"=w166) -> ("error out"=w167:errorcluster)  [unwired: 10 in, 1 out]
      }
      frame "Macro: GUI Stop" {
        # "Cleanups the standalone mode and stop the execution.\nDon't remove 'GUI: Unregister Event', 'GUI: Cleanup Data' and 'Exit'."
        n61 = call <userlib>:"Enqueue.vi"("Queue in"=w171, "States"=string[] ["GUI: Unregister Event", "GUI: Cleanup Data", "Exit"], "Enqueue at Front?(F)"=TRUE, "error in (no error)"=w173) -> ("error out"=w174:errorcluster)  [unwired: 10 in, 1 out]
      }
      frame "--------------- GUI Mode-----------------" {
        # "Not used. category splitter"
      }
      frame "GUI: Initialize Data" {
        w196 = T6."Output Voltage Vs Input Voltage Curve" ("Result Enum")
        w197 = T1."Station Setup" ("Tab Enum")
        w200 = string[][] []  # Test Results[][]
        w210 = T14 {"Measured Input Voltage in V"=[], "Measured Output Voltage in V"=[], "Dropout Voltage in V"=0.0}  # Test Results
        # "Add the front panel controls terminal here and connect them to the bundle structure, So they will be available through data cluster in every case. If the controls and indicators are added to the 'Test Inputs' & 'Test Results' cluster then they are already available in the data cluster since they are typedefs."
        n62 = property on="Run" class="Bool (strict)"(error in=w204, "DisabledEnum"=T17."Enabled" ("Disabled")) -> (error out=w207:errorcluster)  [unwired: 1 in, 1 out]
        n63 = property on="Terminate" class="Bool (strict)"(error in=w207, "DisabledEnum"=T17."Disabled and Grayed Out" ("Disabled")) -> (error out=w203:errorcluster)  [unwired: 1 in, 1 out]
        n64 = property on="Progress" class="Slide (strict)"(error in=w203, "Visible"=FALSE) -> (error out=w202:errorcluster)  [unwired: 1 in, 1 out]
        n65 = Bundle By Name(cluster=w209, "Test Pins"="Test Pins", "Test Inputs"="Test Inputs", "Test Results"=w210, "Test Results[][]"=w200, "Logger Folder Path"="DataLogPath") -> (w195:T16)
        n66 = local write "Tab Enum"(w197) -> ()
        n67 = local write "Tab Control"(w197) -> ()
        n68 = local write "Result Enum"(w196) -> ()
        n69 = local write "Result Tab"(w196) -> ()
        n70 = control-ref of="Result Enum"() -> (w192:refnum<vi>)
        n71 = control-ref of="Customize Sweep Value"() -> (w183:refnum<vi>)
        n72 = control-ref of="Tab Enum"() -> (w180:refnum<vi>)
        n73 = control-ref of="Customize Sweep Value"() -> (w182:refnum<vi>)
        n74 = control-ref of="Advanced Settings"() -> (w181:refnum<vi>)
        n75 = control-ref of="SystemSetup"() -> (w191:refnum<vi>)
        n76 = control-ref of="Dropout Voltage (V)"() -> (w179:refnum<vi>)
        n77 = control-ref of="Nominal Output Voltage (V)"() -> (w190:refnum<vi>)
        n78 = control-ref of="Load Current (A)"() -> (w189:refnum<vi>)
        n79 = control-ref of="Req. Voltage Drop"() -> (w188:refnum<vi>)
        n80 = control-ref of="Start Value (V)"() -> (w186:refnum<vi>)
        n81 = control-ref of="Stop Value (V)"() -> (w185:refnum<vi>)
        n82 = control-ref of="Step Size (V)"() -> (w184:refnum<vi>)
        n83 = control-ref of="Input Voltage (V)"() -> (w187:refnum<vi>)
        n84 = Build Array(w192, w191, w190, w189, w188, w187, w186, w185, w184, w183, w182, w181, w180, w179) -> (w193:refnum<vi>[])
        n85 = Bundle By Name(cluster=w195, "UI Ctls"=w193) -> (w194:T16)
      }
      frame "GUI: Register Event" {
        # "Hidden in UI"
        # "Register for the events from caller."
        n86 = register-events(error in=w216, "Caller Events") -> (reference out=w213:refnum<event-registration>, error out=w214:errorcluster)  [unwired: 1 in]
      }
      frame "GUI: Unregister Event" {
        n87 = Unregister For Events(event registration refnum=w217, error in=w220) -> (error out=w218:errorcluster)
      }
      frame "GUI: Cleanup Data" {
        # "Cleanup the reference or other resources before exiting"
      }
      frame "GUI: Generate Iload" {
        n88 = property on="Step Input" class="Clust (strict)"(error in=w238) -> (error out=w227:errorcluster, "Value"=w237:T20)  [unwired: 1 in, 1 out]
        n89 = Unbundle By Name(w237) -> ("Start Value"=w236:dbl, "Stop Value"=w235:dbl, "Step Size"=w234:dbl)
        n90 = property on="Customize Sweep Value" class="RadioBtnsControl (strict)"(error in=w227) -> (error out=w229:errorcluster, "Value"=w231:enum32{"Item 0", "Item 1"})  [unwired: 1 in, 1 out]
        n91 = call "Get Range Values[].vi"("Start"=w236, "Stop"=w235, "Step Size"=w234) -> ("Values[]"=w230:dbl[])  [unwired: 12 in]
        n92 = case shown="\"Item 1\"" w231 {
          tunnel: w230 -> [w241 w242]
          tunnel: [w241 w244] -> w224
          tunnel: w229 -> [w240 w246]
          tunnel: [w240 w245] -> w228
          frame "Item 0", Default {
            # "Replace Existing"
          }
          frame "Item 1" {
            # "Append to end"
            n93 = property on="Input Voltage (V)" class="Arr (strict)"(error in=w246) -> (error out=w245:errorcluster, "Value"=w243:dbl[])  [unwired: 1 in, 1 out]
            n94 = Insert Into Array(array=w243, new element=w242) -> (w244:dbl[])  [unwired: 1 in]
          }
        }
        n95 = property on="Input Voltage (V)" class="Arr (strict)"(error in=w228, "Value"=w224) -> (error out=w233:errorcluster)  [unwired: 1 in, 1 out]
        n96 = Bundle By Name(cluster=w225, "Test Inputs.Input Voltage in V"=w224) -> (w226:T16)
        n97 = property on="Input Voltage in V" class="Arr (strict)"(error in=w233, "Value"=w224) -> (error out=w232:errorcluster)  [unwired: 1 in, 1 out]
      }
      frame "GUI: Update Measurement Table" {
        n98 = Unbundle By Name(w249) -> ("Test Results.Measured Input Voltage in V"=w254:dbl[], "Test Results.Measured Output Voltage in V"=w252:dbl[])
        n99 = Build Array(w254, w252) -> (w253:dbl[][])
        n100 = Transpose 2D Array(2D array=w253) -> (transposed array=w251:dbl[][])
        n101 = Number To Fractional String(number=w251, precision (6)=i16 5) -> (F-format string=w248:string[][])  [unwired: 2 in]
        "Measured Values" <- w248
        n102 = Bundle By Name(cluster=w249, "Test Results[][]"=w248) -> (w250:T16)
      }
      frame "GUI: Update Cursor Legend" {
        n103 = control-ref of="Dropout Voltage"() -> (w262:refnum<vi>)
        n104 = property class="XYGraph (strict)"(reference=w262, error in=w268) -> (error out=w266:errorcluster, "CrsrList"=w257:T21)  [unwired: 1 out]
        n105 = for {
          tunnel: w257 -> [w299] mode=indexing
          tunnel: [w297] -> w264 if=w296
          tunnel: [w295] -> w258
          i -> [w295]
          # "Check if cursor exist"
          n106 = Unbundle By Name(w299) -> ("Name"=w297:string)
          n107 = Equal?(x=w297, y="Dropout Voltage") -> (x = y?=w296:bool)
        }
        n108 = Unbundle By Name(w261) -> ("Input Voltage_x"=w260:dbl, "Output Voltage_x"=w259:dbl)
        n109 = Empty String/Path?(string/path=w264) -> (empty?=w263:bool)
        n110 = case shown="True" w263 {
          tunnel: w266 -> [w279 w294]
          tunnel: [w278 w293] -> w265
          tunnel: w260 -> [w273 w288]
          tunnel: w259 -> [w272 w287]
          tunnel: w258 -> [w276 _]
          tunnel: w257 -> [w271 w284]
          frame False {
            # "Update existing legend"
            n111 = control-ref of="Dropout Voltage"() -> (w269:refnum<vi>)
            n112 = Index Array(array=w271, index=w276) -> (element=w277:T18)
            n113 = Bundle By Name(cluster=w277, "Position.X"=w273, "Position.Y"=w272, "Allow Drag"=FALSE) -> (w275:T18)
            n114 = Replace Array Subset(array=w271, new element=w275, index=w276) -> (w274:T21)
            n115 = property class="XYGraph (strict)"(reference=w269, error in=w279, "CrsrList"=w274) -> (error out=w278:errorcluster)  [unwired: 1 out]
          }
          frame True {
            # "Create new cursor"
            n116 = Bundle By Name(cluster=T18 {"Name"="", "Color"=0, "Style"=0, "Point Style"=0, "Name Visible"=FALSE, "Allow Drag"=FALSE, "Cursor Mode"=0, "Plot"=0, "Index"=0, "Position"={"X"=0.0, "Y"=0.0}, "X Scale"=0, "Y Scale"=0, "Watch Plots"=[], "Watch All Plots"=FALSE, "Plot Area"=0, "Label Offset"={"X"=0.0, "Y"=0.0}} ("element"), "Name"="Dropout Voltage", "Color"=u32 11776947, "Style"=u8 8, "Point Style"=u8 6, "Position.X"=w288, "Position.Y"=w287) -> (w283:T18)
            n117 = Array Size(array=w284) -> (size(s)=w282:i32)
            n118 = Insert Into Array(array=w284, index=w282, new element=w283) -> (w281:T21)
            n119 = control-ref of="Dropout Voltage"() -> (w280:refnum<vi>)
            n120 = property class="XYGraph (strict)"(reference=w280, error in=w294, "CrsrList"=w281, "Cursor.LineStyle"=u8 1 ("Cursor.Line Style")) -> (error out=w293:errorcluster)  [unwired: 1 out]
          }
        }
      }
      frame "GUI: Update Cursor Label" {
        w330 = T22 {"Name"="", "Color"=9934743, "Style"=0, "Point Style"=0, "Name Visible"=TRUE, "Allow Drag"=FALSE, "Annotation Mode"=0, "Plot"=0, "Index"=0, "Position"={"X"=0.0, "Y"=0.0}, "X Scale"=0, "Y Scale"=0, "Show Arrow"=FALSE, "Lock Name"=FALSE, "Plot Area"=0, "Label Offset"={"X"=0.0, "Y"=0.0}} ("new element/subarray")
        # "Forcedraw to update increments"
        # "Adding Scale Increment to move Annotation in appropriate position"
        # "X label is placed at the bottom just above X axis\nY label is placed to the right of Y axis"
        n121 = Unbundle By Name(w329) -> ("Input Voltage_x"=w320:dbl, "Output Voltage_x"=w319:dbl)
        n122 = control-ref of="Dropout Voltage"() -> (w311:refnum<vi>)
        n123 = invoke class="XYGraph (strict)" method="ForceRedraw"(reference=w311, error in=w337) -> (reference out=w310:refnum<vi>, error out=w312:errorcluster)  [unwired: 1 in, 1 out]
        n124 = property class="XYGraph (strict)"(reference=w310, error in=w312) -> (reference out=w327:refnum<vi>, error out=w328:errorcluster, "YScale.Minimum"=w324:dbl, "XScale.Minimum"=w321:dbl, "XScale.Increment"=w322:dbl, "YScale.Increment"=w323:dbl)
        n125 = Multiply(x=w322, y=2.0) -> (x*y=w303:dbl)
        n126 = Add(x=w321, y=w303) -> (x+y=w314:dbl)
        n127 = Divide(x=w323, y=2.0) -> (x/y=w325:dbl)
        n128 = Multiply(x=w322, y=1.5) -> (x*y=w301:dbl)
        n129 = Add(x=w325, y=w319) -> (x+y=w313:dbl)
        n130 = Add(x=w324, y=w323) -> (x+y=w315:dbl)
        n131 = Number To Fractional String(number=w320, precision (6)=i16 5) -> (F-format string=w308:string)  [unwired: 2 in]
        n132 = Number To Fractional String(number=w319, precision (6)=i16 5) -> (F-format string=w305:string)  [unwired: 2 in]
        n133 = Add(x=w320, y=w301) -> (x+y=w316:dbl)
        n134 = Concatenate Strings("Input Voltage-x: " ("string"), w308) -> (w307:string)
        n135 = Concatenate Strings("Output Voltage-x: " ("string"), w305) -> (w304:string)
        n136 = Bundle By Name(cluster=w330, "Name"=w307, "Position.X"=w316, "Position.Y"=w315) -> (w332:T22)
        n137 = Bundle By Name(cluster=w330, "Name"=w304, "Position.X"=w314, "Position.Y"=w313) -> (w331:T22)
        n138 = Insert Into Array(array=T19 [] ("Annotation List"), new element #1=w332, new element #2=w331) -> (w333:T19)  [unwired: 1 in]
        n139 = property class="XYGraph (strict)"(reference=w327, error in=w328, "AnntList"=w333) -> (error out=w335:errorcluster)  [unwired: 1 out]
      }
      frame "GUI: Get Logger File Path" {
        n140 = Unbundle By Name(w338) -> ("Logger Folder Path"=w345:path)
        n141 = call <vilib>:"Check if File or Folder Exists.vi"("error in (no error)"=w341, "path"=w345) -> ("error out"=w344:errorcluster, "file or folder exists?"=w343:bool, "dup path"=w342:path)  [unwired: 7 in]
        n142 = case shown="True" w343 {
          tunnel: [w348 w350] -> w340
          tunnel: w344 -> [w348 w350]
          tunnel: w338 -> [w347 w353]
          tunnel: [w347 w352] -> w339
          tunnel: w342 -> [_ w349]
          frame False {
          }
          frame True {
            n143 = Bundle By Name(cluster=w353, "Valid Logger Path?"=TRUE ("Valid Logger path?"), "Logger File Path"=w349) -> (w352:T16)
          }
        }
      }
      frame "GUI: Log" {
        n144 = Unbundle By Name(w360) -> ("Valid Logger Path?"=w354:bool, "Test Inputs"=w356:T8, "Test Results"=w357:T14, "Logger File Path"=w355:path)
        n145 = case shown="True" w354 {
          tunnel: [w362 w367] -> w359
          tunnel: w358 -> [w362 w366]
          tunnel: w357 -> [_ w365]
          tunnel: w356 -> [_ w364]
          tunnel: w355 -> [_ w363]
          frame False {
          }
          frame True {
            n146 = call "Log Data.vi"("Test Inputs"=w364, "Test Results"=w365, "DataLogger File Path"=w363, "error in (no error)"=w366) -> ("error out"=w367:errorcluster)  [unwired: 11 in]
          }
        }
      }
      frame "GUI: Set Busy" {
        n147 = Unbundle By Name(w368) -> ("UI Ctls"=w374:refnum<vi>[])
        n148 = for {
          tunnel: [w379] -> w375 mode=indexing
          tunnel: w369 -> [w380]
          tunnel: w374 -> [w378] mode=indexing
          tunnel: T17."Disabled and Grayed Out" ("Disabled") -> [w377]
          n149 = property class="Ctl"(reference=w378, error in=w380, "DisabledEnum"=w377) -> (error out=w379:errorcluster)  [unwired: 1 out]
        }
        n150 = Merge Errors(w375) -> (w372:errorcluster)
        n151 = call "Defer Front Panel.vi"("Defer Front Panel?"=TRUE, "error in"=w372) -> ("error out"=w370:errorcluster)  [unwired: 13 in]
      }
      frame "GUI: Unset Busy" {
        n152 = Unbundle By Name(w382) -> ("UI Ctls"=w387:refnum<vi>[])
        n153 = for {
          tunnel: [w392] -> w388 mode=indexing
          tunnel: w381 -> [w393]
          tunnel: w387 -> [w391] mode=indexing
          tunnel: T17."Enabled" ("Disabled") -> [w390]
          n154 = property class="Ctl"(reference=w391, error in=w393, "DisabledEnum"=w390) -> (error out=w392:errorcluster)  [unwired: 1 out]
        }
        n155 = Merge Errors(w388) -> (w385:errorcluster)
        n156 = call "Defer Front Panel.vi"("Defer Front Panel?"=FALSE, "error in"=w385) -> ("error out"=w383:errorcluster)  [unwired: 13 in]
      }
      frame "------------ TerminationMonitor -----------" {
        # "Not used. category splitter"
      }
      frame "TerminationMonitor: Start" {
        # "Termination Monitor monitors the execution of the caller. Use Termination Monitor Status to get the termination status. If the caller is terminating, stop the test procedure, cleanup and stop."
        n157 = Unbundle By Name(w399) -> ("Termination Monitor Info.Caller Information"=w398:T11)
        n158 = call <userlib>:"Termination Monitor Start.vi"("Caller Information"=w398, "error in (no error)"=w401) -> ("Termination Monitor Info out"=w397:T15, "error out"=w402:errorcluster)  [unwired: 12 in]
        n159 = Bundle By Name(cluster=w399, "Termination Monitor Info"=w397) -> (w400:T16)
      }
      frame "TerminationMonitor: Stop" {
        n160 = Unbundle By Name(w406) -> ("Termination Monitor Info"=w405:T15)
        n161 = call <userlib>:"Termination Monitor Stop.vi"("Status Info in"=w405, "error in (no error)"=w408) -> ("Status Info out"=w404:T15, "error out"=w409:errorcluster)  [unwired: 12 in]
        n162 = Bundle By Name(cluster=w406, "Termination Monitor Info"=w404) -> (w407:T16)
      }
      frame "------------ Automation Mode -----------" {
        # "Not used. category splitter"
      }
      frame "Test: Start" {
        # "Reinitialize/Reset/Update the data from the UI to the data cluster so that the data will be considered for the test procedure.\nReset the Test Results."
        n163 = local read "DataLogPath"() -> (w414:path)
        n164 = local read "Test Inputs"() -> (w429:T8)
        n165 = local read "Test Pins"() -> (w415:T7)
        n166 = property on="Run" class="Bool (strict)"(error in=w426, "DisabledEnum"=T17."Disabled and Grayed Out" ("Disabled")) -> (error out=w424:errorcluster)  [unwired: 1 in, 1 out]
        n167 = Bundle By Name(cluster=w430, "Test Pins"=w415, "Test Inputs"=w429, "Test Results"=T14 {"Measured Input Voltage in V"=[], "Measured Output Voltage in V"=[], "Dropout Voltage in V"=0.0}, "Logger Folder Path"=w414) -> (w419:T16)
        n168 = property on="Terminate" class="Bool (strict)"(error in=w424, "DisabledEnum"=T17."Enabled" ("Disabled")) -> (error out=w421:errorcluster)  [unwired: 1 in, 1 out]
        n169 = Unbundle By Name(w419) -> ("Test Inputs.Input Voltage in V"=w418:dbl[])
        n170 = Array Size(array=w418) -> (size(s)=w417:i32)
        n171 = property on="Progress" class="Slide (strict)"(error in=w421, "Visible"=TRUE, "Scale.Maximum"=w417, "Value"=0 ("Progress")) -> (error out=w420:errorcluster)  [unwired: 1 in, 1 out]
      }
      frame "Test: Prepare DCPower" {
        # "Set load current as Initial current\nSet first index of Input Voltage as initial Voltage"
        n172 = Unbundle By Name(w440) -> ("Test Pins.Set Load Current"=w432:string, "Test Inputs.Load Current in A"=w433:dbl, "Test Inputs.Advance Setting.Prepare.Load SMU Output Function"=w434:T10, "Test Pins.Set Input Voltage"=w438:string, "Test Inputs.Input Voltage in V"=w437:dbl[])
        n173 = Index Array(array=w437) -> (element=w431:dbl)  [unwired: 1 in]
        n174 = call "Prepare Source.vi"("Set Vin"=w438, "Initial Voltage Level (V)"=w431, "error in (no error)"=w439) -> ("error out"=w436:errorcluster)  [unwired: 12 in]
        n175 = call "Prepare Load.vi"("PinName"=w432, "Load Current Level (A)"=w433, "error in (no error)"=w436, "Load Output Function"=w434) -> ("error out"=w435:errorcluster)  [unwired: 11 in]
      }
      frame "Test: Prepare DMM" {
        w454 = 1 items=["DC Volts"=1, "AC Volts"=2, "DC Current"=3, "AC Current"=4, "2-Wire Resistance"=5, "4-Wire Resistance"=101, "Frequency"=104, "Period"=105, "AC Volts DC Coupled"=1001, "Diode"=1002, "Waveform Voltage"=1003, "Waveform Current"=1004, "Capacitance"=1005, "Inductance"=1006, "Temperature"=108] ("Configuration:Function")
        w455 = 1 items=["DC Volts"=1, "AC Volts"=2, "DC Current"=3, "AC Current"=4, "2-Wire Resistance"=5, "4-Wire Resistance"=101, "Frequency"=104, "Period"=105, "AC Volts DC Coupled"=1001, "Diode"=1002, "Waveform Voltage"=1003, "Waveform Current"=1004, "Capacitance"=1005, "Inductance"=1006, "Temperature"=108] ("Configuration:Function")
        # "Adding abort.vi to stop prev acquisition"
        n176 = Unbundle By Name(w458) -> ("Test Pins.Measure Input Voltage"=w448:string, "Test Pins.Measure Output Voltage"=w449:string)
        n177 = call "Pin Name to Reference.vim"("Pin Name"=w449, "type"=refnum<k15> refnum ("instrument handle"), "error in (no error)"=w457) -> ("Reference"=w446:refnum<k15>, "error out"=w456:errorcluster)  [unwired: 7 in, 4 out]
        n178 = call <instrlib>:"niDMM Abort.vi"("error in (no error)"=w456, "instrument handle"=w446) -> ("error out"=w447:errorcluster, "instrument handle out"=w445:refnum<k15>)  [unwired: 8 in]
        n179 = property class="niDMM"(reference=w445, error in=w447, "Function"=w455) -> (error out=w451:errorcluster)  [unwired: 1 out]
        n180 = call "Pin Name to Reference.vim"("Pin Name"=w448, "type"=refnum<k15> refnum ("instrument handle"), "error in (no error)"=w451) -> ("Reference"=w443:refnum<k15>, "error out"=w453:errorcluster)  [unwired: 7 in, 4 out]
        n181 = call <instrlib>:"niDMM Abort.vi"("error in (no error)"=w453, "instrument handle"=w443) -> ("error out"=w444:errorcluster, "instrument handle out"=w442:refnum<k15>)  [unwired: 8 in]
        n182 = property class="niDMM"(reference=w442, error in=w444, "Function"=w454) -> (error out=w450:errorcluster)  [unwired: 1 out]
      }
      frame "Test: Set Load Current" {
        n183 = Unbundle By Name(w465) -> ("Test Pins.Set Load Current"=w461:string, "Test Inputs.Load Current in A"=w462:dbl, "Test Inputs.Advance Setting.Prepare.Load SMU Output Function"=w463:T10)
        n184 = call "Set Load Current.vi"("PinName"=w461, "current level"=w462, "error in (no error)"=w466, "OutputFunction"=w463) -> ("error out"=w464:errorcluster)  [unwired: 11 in]
      }
      frame "Test: Sweep Over Voltage" {
        n185 = Unbundle By Name(w487) -> ("Termination Monitor Info"=w483:T15, "Test Inputs.Advance Setting.Stimulus and Measure.Loop Delay in milliseconds"=w470:u32, "Test Pins.Set Input Voltage"=w468:string, "Test Inputs.Input Voltage in V"=w471:dbl[], "Test Pins.Measure Input Voltage"=w475:string, "Test Pins.Measure Output Voltage"=w476:string)
        n186 = call "Pin Name to Reference.vim"("Pin Name"=w476, "type"=refnum<k15> refnum ("instrument handle"), "error in (no error)"=w479) -> ("Reference"=w473:refnum<k15>, "error out"=w477:errorcluster)  [unwired: 7 in, 4 out]
        n187 = call "Pin Name to Reference.vim"("Pin Name"=w475, "type"=refnum<k15> refnum ("instrument handle"), "error in (no error)"=w477) -> ("Reference"=w474:refnum<k15>, "error out"=w469:errorcluster)  [unwired: 7 in, 4 out]
        n188 = for {
          shift-right: [w504] -> w484
          shift-left: w469 -> [w491]
          shift-right: [w502] -> w472
          shift-left: w483 -> [w503]
          tunnel: [w497] -> w482 mode=indexing
          tunnel: [w498] -> w481 mode=indexing
          tunnel: w471 -> [w489] mode=indexing
          tunnel: w474 -> [w496]
          tunnel: w473 -> [w495]
          tunnel: w470 -> [w492]
          tunnel: w468 -> [w488]
          i -> [w500]
          stop <- w501 stop-if-true
          n189 = call "Set Source.vi"("Set Vin"=w488, "Vin in V"=w489, "error in (no error)"=w491) -> ("error out"=w490:errorcluster)  [unwired: 12 in]
          n190 = call "Stall Data Flow.vim"("value in"=w490, "milliseconds to wait"=w492) -> ("value out"=w493:errorcluster)  [unwired: 1 out]
          n191 = call <instrlib>:"niDMM Read.vi"("error in (no error)"=w493, "instrument handle"=w496) -> ("error out"=w494:errorcluster, "Measurement"=w498:dbl)  [unwired: 7 in, 1 out]
          n192 = call <instrlib>:"niDMM Read.vi"("error in (no error)"=w494, "instrument handle"=w495) -> ("error out"=w499:errorcluster, "Measurement"=w497:dbl)  [unwired: 7 in, 1 out]
          n193 = call <userlib>:"Termination Monitor Status.vi"("Termination Monitor Info in"=w503, "error in (no error)"=w499) -> ("Termination Monitor Info out"=w502:T15, "Terminating?"=w501:bool, "error out"=w504:errorcluster)  [unwired: 11 in]
          "Progress" <- w500
        }
        n194 = Bundle By Name(cluster=w487, "Termination Monitor Info"=w472, "Test Results.Measured Input Voltage in V"=w481, "Test Results.Measured Output Voltage in V"=w482) -> (w486:T16)
      }
      frame "Test: Cleanup DCPower" {
        n195 = Unbundle By Name(w522) -> ("Test Pins.Set Input Voltage"=w517:string, "Test Pins.Set Load Current"=w519:string)
        n196 = call "Pin Name to Reference.vim"("Pin Name"=w519, "type"=refnum<k15> refnum ("instrument handle"), "error in (no error)"=w520) -> ("Reference"=w510:refnum<k15>, "error out"=w509:errorcluster)  [unwired: 7 in, 4 out]
        n197 = call <instrlib>:"niDCPower Configure Output Enabled.vi"("error in (no error)"=w509, "output enabled"=FALSE, "instrument handle"=w510) -> ("error out"=w515:errorcluster, "instrument handle out"=w507:refnum<k15>)  [unwired: 7 in]
        n198 = call <instrlib>:"niDCPower Abort With Channels.vi"("error in (no error)"=w515, "instrument handle"=w507) -> ("error out"=w508:errorcluster)  [unwired: 8 in, 1 out]
        n199 = call "Pin Name to Reference.vim"("Pin Name"=w517, "type"=refnum<k15> refnum ("instrument handle"), "error in (no error)"=w508) -> ("Reference"=w512:refnum<k15>, "error out"=w516:errorcluster)  [unwired: 7 in, 4 out]
        n200 = call <instrlib>:"niDCPower Configure Output Enabled.vi"("error in (no error)"=w516, "output enabled"=FALSE, "instrument handle"=w512) -> ("error out"=w514:errorcluster, "instrument handle out"=w505:refnum<k15>)  [unwired: 7 in]
        n201 = call <instrlib>:"niDCPower Abort With Channels.vi"("error in (no error)"=w514, "instrument handle"=w505) -> ("error out"=w506:errorcluster)  [unwired: 8 in, 1 out]
      }
      frame "Test: Cleanup DMM" {
        n202 = Unbundle By Name(w535) -> ("Test Pins.Measure Input Voltage"=w530:string, "Test Pins.Measure Output Voltage"=w532:string)
        n203 = call "Pin Name to Reference.vim"("Pin Name"=w532, "type"=refnum<k15> refnum ("instrument handle"), "error in (no error)"=w533) -> ("Reference"=w526:refnum<k15>, "error out"=w528:errorcluster)  [unwired: 7 in, 4 out]
        n204 = call <instrlib>:"niDMM Abort.vi"("error in (no error)"=w528, "instrument handle"=w526) -> ("error out"=w527:errorcluster)  [unwired: 8 in, 1 out]
        n205 = call "Pin Name to Reference.vim"("Pin Name"=w530, "type"=refnum<k15> refnum ("instrument handle"), "error in (no error)"=w527) -> ("Reference"=w524:refnum<k15>, "error out"=w529:errorcluster)  [unwired: 7 in, 4 out]
        n206 = call <instrlib>:"niDMM Abort.vi"("error in (no error)"=w529, "instrument handle"=w524) -> ("error out"=w525:errorcluster)  [unwired: 8 in, 1 out]
      }
      frame "Test: Calculate Dropout Voltage" {
        # "Input Voltage(nominal voltage – Required voltage drop at output voltage)  - Output Voltage(nominal voltage – Required voltage drop at output voltage)"
        n207 = Unbundle By Name(w549) -> ("Test Results.Measured Input Voltage in V"=w542:dbl[], "Test Results.Measured Output Voltage in V"=w540:dbl[], "Test Inputs.Nominal Output Voltage in V"=w545:dbl, "Test Inputs.Required Vout drop"=w544:dbl)
        n208 = Subtract(x=w545, y=w544) -> (x-y=w537:dbl)
        n209 = call "Sort Voltage.vi"("Input Voltage"=w542, "Output Voltage"=w540) -> ("Sorted Input Voltage"=w541:dbl[], "Sorted Output Voltage"=w539:dbl[])  [unwired: 12 in]
        n210 = Threshold 1D Array(2:w537, 3:w539) -> (0:w546:dbl)  [unwired: 1 in]
        n211 = Interpolate 1D Array(1:w546, 2:w541) -> (0:w538:dbl)
        n212 = Subtract(x=w538, y=w537) -> (x-y=w543:dbl)
        n213 = Bundle By Name(cluster=w549, "Input Voltage_x"=w538, "Test Results.Dropout Voltage in V"=w543, "Output Voltage_x"=w537) -> (w548:T16)
      }
      frame "Test: Update UI" {
        # "If you want to update more indicators in the front panel do it here. It is efficient to update the UI in one case rather than in several cases. Also, it is a good practice to store the results in the data cluster in an efficient format and then get the data from data cluster and update the UI, in that way we could have the front panel independent of how we manipulate the data."
        n214 = Unbundle By Name(w557) -> ("Test Results.Measured Input Voltage in V"=w555:dbl[], "Test Results"=w554:T14, "Test Results.Dropout Voltage in V"=→"Dropout Voltage (V)":dbl)
        "Test Results" <- w554
        n215 = Unbundle By Name(w554) -> ("Measured Output Voltage in V"=w553:dbl[])
        n216 = Bundle("Measured Input Voltage in V"=w555, "Measured Output Voltage in V"=w553) -> (→"Dropout Voltage":T23)  [unwired: 1 in]
      }
      frame "Test: End" {
        # "End of the Test Procedure. Do cleanup of resources or references."
        n217 = property on="Run" class="Bool (strict)"(error in=w564, "Value"=FALSE ("Run"), "DisabledEnum"=T17."Enabled" ("Disabled")) -> (error out=w567:errorcluster)  [unwired: 1 in, 1 out]
        n218 = property on="Terminate" class="Bool (strict)"(error in=w567, "DisabledEnum"=T17."Disabled and Grayed Out" ("Disabled")) -> (error out=w562:errorcluster)  [unwired: 1 in, 1 out]
        n219 = property on="Progress" class="Slide (strict)"(error in=w562, "Visible"=FALSE, "Value"=0 ("Progress")) -> (error out=w561:errorcluster)  [unwired: 1 in, 1 out]
      }
      frame "---------------------Misc-----------------------" {
      }
      frame "Error" {
        # "Handle the error and make sure to clear the error."
        n220 = Unbundle By Name(w576) -> ("Termination Monitor Info.Caller Information.Mode"=w575:T12)
        n221 = case shown="\"MeasurementSuite\"" w575 {
          tunnel: w579 -> [w583 w588 w590]
          tunnel: [w581 w585 w589] -> w577
          tunnel: [_ TRUE _] -> w574
          tunnel: w573 -> [_ w586 _]
          frame "Standalone" {
            w580 = T24 2 items=["no dialog", "OK message", "continue or stop message", "OK message + warnings", "continue/stop + warnings"] ("type of dialog (OK msg:1)")
            n222 = call <vilib>:"General Error Handler.vi"("type of dialog (OK msg:1)"=w580, "error in (no error)"=w583) -> ("error out"=w582:errorcluster)  [unwired: 9 in, 4 out]
            n223 = call <vilib>:"Clear Errors.vi"("error in (no error)"=w582) -> ("error out"=w581:errorcluster)  [unwired: 5 in, 1 out]
          }
          frame "Automation" {
            n224 = call <userlib>:"Release.vi"("Queue in"=w586) -> ("Error Out"=w584:errorcluster)  [unwired: 14 in]
            n225 = Merge Errors(w588, w584) -> (w585:errorcluster)
          }
          frame "MeasurementSuite" {
            n226 = property on="ErrorOccured" class="Clust (strict)"("Val(Sgnl)"=w590) -> (error out=w589:errorcluster)  [unwired: 2 in, 1 out]
          }
        }
      }
      frame "Exit" {
        # "Last case called before stopping the execution. \nError occured in this state will not be captured by Error state."
        n227 = call <userlib>:"Release.vi"("Queue in"=w596, "Error In"=w597) -> ("Error Out"=w592:errorcluster)  [unwired: 13 in]
        n228 = property on="Progress" class="Slide (strict)"(error in=w592, "Visible"=TRUE) -> (error out=w591:errorcluster)  [unwired: 1 in, 1 out]
      }
    }
  }
  "error out" <- w4
  "Header" <- "Dropout Voltage" ("Header")
